vi "Actor Core.vi"(8 "error in":errorcluster, 11 "Right Panel in":refnum<class "ManualButtons.lvclass">) -> (0 "error out":errorcluster, 3 "Actor out":refnum<class "Actor.lvclass">)   [LabVIEW 2023, in "ManualButtons.lvlib" / "ManualButtons.lvclass"]
doc: "Base Class for the right subpanel.\nThis provides the basic implementation for show/hide operations.\n\nancestor classes should override this, but maintain proportions."
uses:
  Library/ManualButtons.lvclass
  builds/Framework/Actor Framework.lvlibp/1abvi3w/vi.lib/ActorFramework/Actor/Actor.lvclass
  builds/Main/Docking.lvlibp/Right Panel/RightDock.lvclass
  builds/Framework/Engine.lvlibp/Engine/Library/Engine.lvclass
  C:/Users/Public/Documents/Development/builds/Framework/Engine.lvlibp/Engine/Library/Engine.lvclass
panel:
  in  "Restore Defaults":bool
  in  "New Log":bool
  in  "Comments":bool
  in  "New Test Name":bool
  in  "PowerOff":bool
  in  "PowerOn":bool
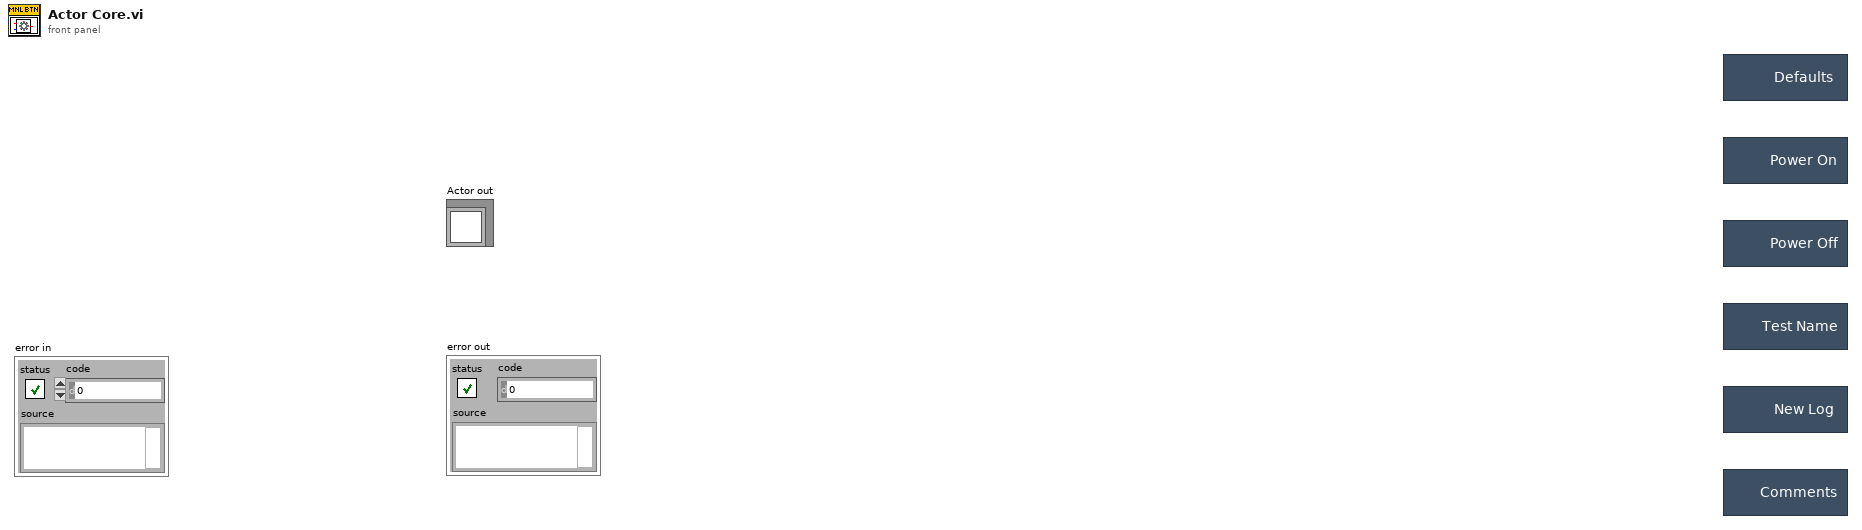
[diagram p1: front panel]
types:
  T1 = cluster{"Pnl Actor":refnum<event-registration>, "Event Registration Refnum":refnum<event-registration>}
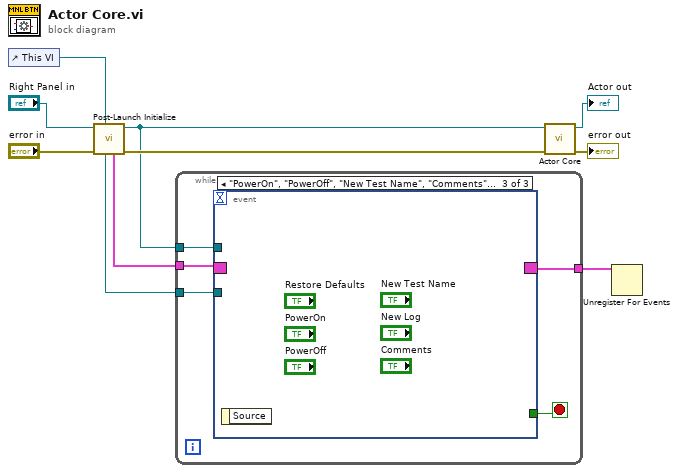
[diagram p0: block diagram]
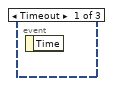
[diagram p2: hidden frame]
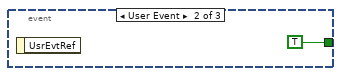
[diagram p3: hidden frame]
diagram:
  n1 = control-ref of="This VI"() -> (w1:refnum<vi>)
  n2 = call "Post-Launch Initialize.vi"("GUI Reference"=w1, "error in (no error)"="error in", "Engine in"="Right Panel in") -> ("error out"=w7:errorcluster, "Engine out"=w3:refnum<class "ManualButtons.lvclass">, "Registered Events"=w5:T1, "Self Enqueuer"=w4:refnum<class "Message Enqueuer.lvclass">)  [unwired: 5 in]
  n3 = while {
    tunnel: w5 -> [w14]
    tunnel: w4 -> [w12]
    tunnel: w3 -> [w13]
    tunnel: [w15] -> w2
    stop <- w11 stop-if-true
    n4 = event shown="[2] \"PowerOn\", \"PowerOff\", \"New Test Name\", \"Comments\", \"New Log\", \"Restore Defaults\": Value Change" {
      selector: w14 -> [_ _ _]
      dyn-events: [_ _ _] -> w15
      timeout: _ -> [_ _ _]
      tunnel: w13 -> [_ _ _]
      tunnel: w12 -> [_ _ _]
      tunnel: [_ TRUE _] -> w11
      event Timeout {
        n5 = event-data() -> ()  [unwired: 1 in, 1 out]
      }
      event User Event {
        n6 = event-data() -> ()  [unwired: 1 in, 1 out]
      }
      event "PowerOn", "PowerOff", "New Test Name", "Comments", "New Log", "Restore Defaults": Value Change {
        n7 = event-data() -> ()  [unwired: 1 in, 1 out]
      }
    }
  }
  n8 = call-parent "Actor Core.vi"("error in"=w7, "Right Panel in"=w3) -> ("error out"=→"error out":errorcluster, "Actor out"=→"Actor out":refnum<class "Actor.lvclass">)  [unwired: 8 in]
  n9 = Unregister For Events(event registration refnum=w2) -> ()  [unwired: 1 in, 1 out]
